vi "MeasAction.vi"(8 "error in (no error)":errorcluster caption="entrée d'erreur (pas d'erreur)", 9 "CurvePointIndex":i32, 10 "AllPointIndex":i32, 11 "InstrClassIn":refnum<class "ThorPM100A.lvclass"> caption="DNL_LabVIEW Object in") -> (0 "error out":errorcluster caption="sortie d'erreur", 2 "MeasDatOut":dbl[](array[numeric]), 3 "InstrClassOut":refnum<class "ThorPM100A.lvclass"> caption="DNL_LabVIEW Object out")   [LabVIEW 2019, in "ThorPM100A.lvclass"]
uses:
  ThorPM100A.lvclass
  C:/Programmes Labview/LabScanV1A/DevicesClass/BaseDevice/BaseDevice.lvclass
  ThorPM100A.lvclass/ThorPM100A.ctl
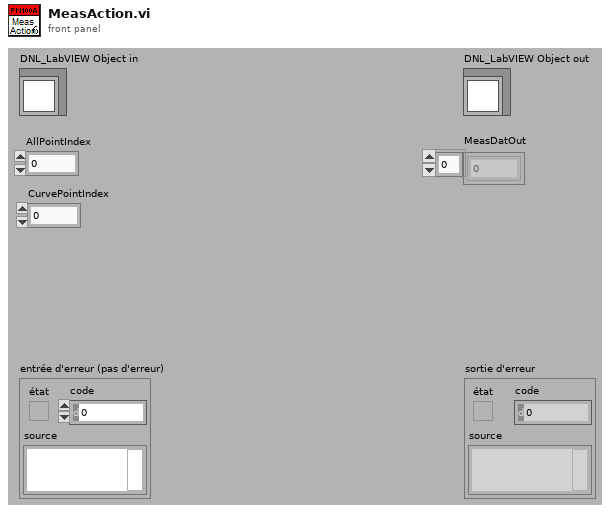
[diagram p1: front panel]
types:
  T1 = typedef "ThorPM100A.lvclass/ThorPM100A_Func.ctl" = enum16{"Read Power (mW)"}
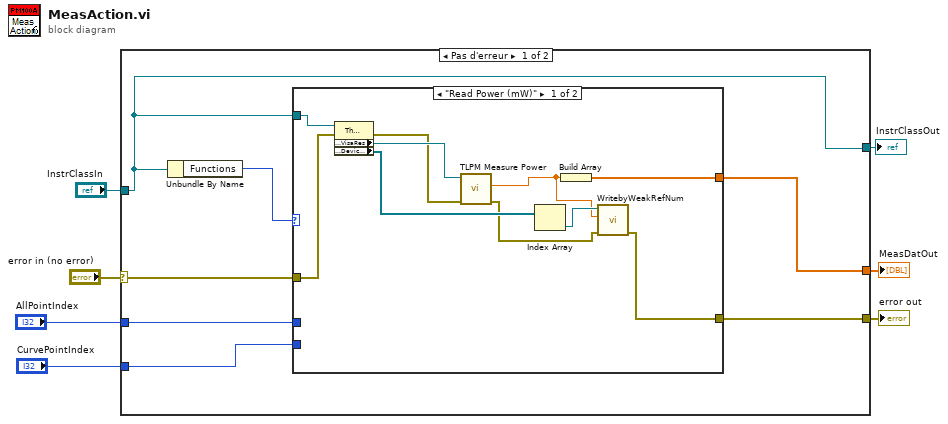
[diagram p0: block diagram]
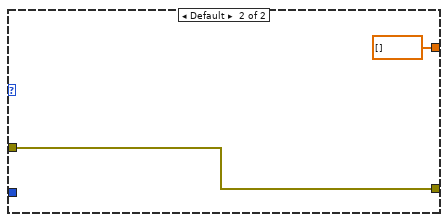
[diagram p2: hidden frame]
diagram:
  n1 = case shown="Pas d'erreur" "error in (no error)" {
    selector: "error in (no error)" -> [w10 w27]
    tunnel: "InstrClassIn" -> [w8 w28]
    tunnel: [w8 w28] -> w5
    tunnel: "AllPointIndex" -> [w14 _]
    tunnel: [w13 w27] -> w3
    tunnel: [w12 _] -> w2
    tunnel: "CurvePointIndex" -> [w9 _]
    frame No Error {
      n2 = Unbundle By Name(w8) -> ("Functions"=w11:T1)
      n3 = case shown="\"Read Power (mW)\"" w11 {
        tunnel: w14 -> [_ _]
        tunnel: [w16 w25] -> w13
        tunnel: [w20 dbl[] [] ("Outputs")] -> w12
        tunnel: w10 -> [w23 w25]
        tunnel: w9 -> [_ _]
        tunnel: w8 -> [w24 _]
        frame "Read Power (mW)" {
          n4 = property class="ThorPM100A.lvclass"(reference=w24, error in=w23) -> (error out=w21:errorcluster, "Accessor:VisaRes"=w22:refnum<visa-resource-name>, "Accessor:DeviceCtrl"=w19:refnum<vi>[])  [unwired: 1 out]
          n5 = call <instrlib>:"TLPM Measure Power.vi"("error in (no error)"=w21, "instrument handle"=w22) -> ("error out"=w17:errorcluster, "Power"=w15:dbl)  [unwired: 7 in, 1 out]
          n6 = Index Array(array=w19) -> (element=w18:refnum<vi>)  [unwired: 1 in]
          n7 = Build Array(w15) -> (w20:dbl[])
          n8 = call <userlib>:"WritebyWeakRefNum.vi"("error in"=w17, "Valeur"=w15, "Control Ref"=w18) -> ("error out"=w16:errorcluster)  [unwired: 8 in]
        }
        frame Default {
        }
      }
    }
    frame Error {
    }
  }
  "error out" <- w3
  "InstrClassOut" <- w5
  "MeasDatOut" <- w2
